vi "Read Enable Output Command (Single).vi"(8 "error in":errorcluster, 9 "Channel Index":i32=1, 11 "Cycler in":refnum<class "Cycler.lvclass">) -> (0 "error out":errorcluster, 1 "Changed or First Call?":bool, 2 "Enable Output":bool, 3 "Cycler out":refnum<class "Cycler.lvclass">)   [LabVIEW 2023, in "Cycler.lvclass"]
uses:
  Cycler.lvclass
  Cycler.lvclass/Cycler.ctl
  <vilib>/ADAS Replay HIL/Channels/Tag Wrapper/Tag Wrapper.lvlib
  <vilib>/ADAS Replay HIL/Channels/Tag Wrapper/Polymorphic/Read Channel (Boolean).vi
  c7b580bb-7e3f-4bc5-b721-470854a20720.vi
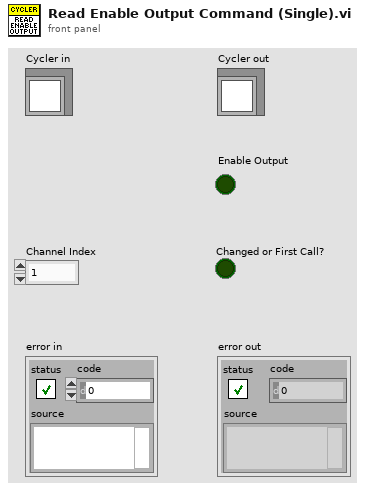
[diagram p1: front panel]
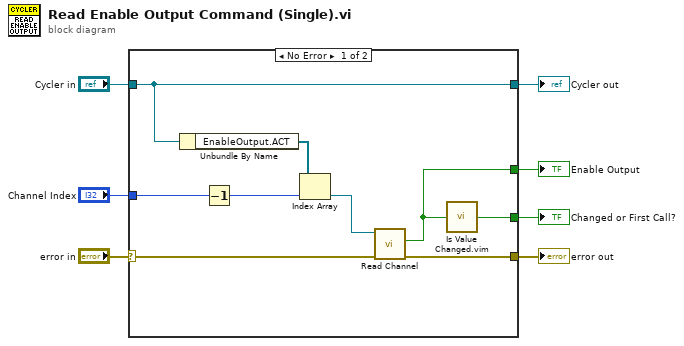
[diagram p0: block diagram]
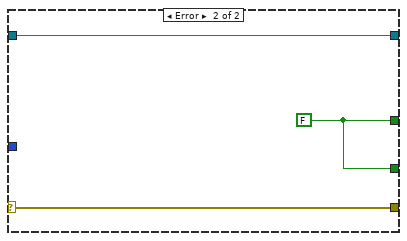
[diagram p2: hidden frame]
diagram:
  n1 = case shown="No Error" "error in" {
    selector: "error in" -> [w15 w18]
    tunnel: [w14 w18] -> w6
    tunnel: [w16 w19] -> w4
    tunnel: "Cycler in" -> [w16 w19]
    tunnel: [w9 w17] -> w3
    tunnel: "Channel Index" -> [w11 _]
    tunnel: [w8 w17] -> w1
    frame No Error {
      n2 = Unbundle By Name(w16) -> ("EnableOutput.ACT"=w13:refnum<k21>[])
      n3 = Decrement(x=w11) -> (x-1=w10:i32)
      n4 = Index Array(array=w13, index=w10) -> (element=w12:refnum<k21>)
      n5 = call-poly <vilib>:"Read Channel.vi"("error in"=w15, "ADAS HIL Channel in"=w12) -> ("error out"=w14:errorcluster, "Value out"=w9:bool)  [unwired: 6 in, 2 out]
      n6 = call "Is Value Changed.vim"("value"=w9) -> ("changed or first call?"=w8:bool)
    }
    frame Error {
      w17 = FALSE ("Value out")
    }
  }
  "error out" <- w6
  "Cycler out" <- w4
  "Enable Output" <- w3
  "Changed or First Call?" <- w1
